vi "XML Script - Structure.vi"   [LabVIEW 2017]
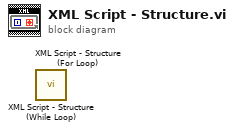
[diagram p0: block diagram]
diagram:
  n1 = call <vilib>:"XML Script - Structure (While Loop).vi"() -> ()  [unwired: 10 in, 2 out]
  n2 = call <vilib>:"XML Script - Structure (For Loop).vi"() -> ()  [unwired: 10 in, 2 out]
